vi "Lift and Clamp Test.vi"() -> ()   [LabVIEW 2014]
panel:
  in  "Clamp Direction":enum16{"Stop", "In", "Out"}(ring)
  out "Lift Encoder":T1
  in  "Lift Direction":enum16{"Stop", "Up", "Down"}(ring)
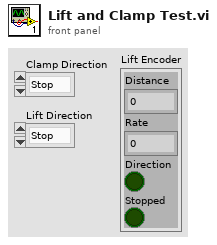
[diagram p1: front panel]
types:
  T1 = cluster{"Distance":dbl, "Rate":dbl, "Direction":bool, "Stopped":bool}
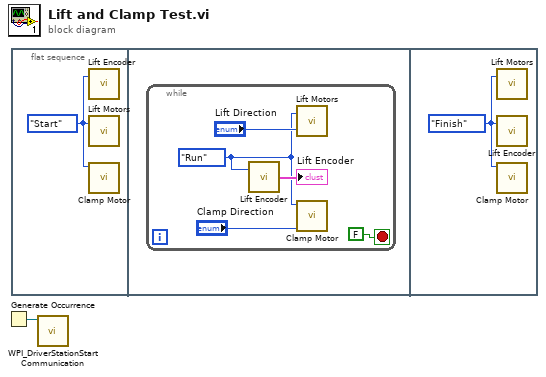
[diagram p0: block diagram]
diagram:
  n1 = Generate Occurrence() -> (w1:refnum<k4>)
  n2 = flat-sequence {
    frame #0 {
      w2 = enum8{"Start", "Run", "Finish"}."Start" ("Mode")
      n3 = call "Lift Encoder.vi"("Mode"=w2) -> ()  [unwired: 1 in, 1 out]
      n4 = call "Lift Motors.vi"("Mode"=w2) -> ()  [unwired: 2 in]
      n5 = call "Clamp Motor.vi"("Mode"=w2) -> ()  [unwired: 3 in]
    }
    frame #1 {
      n6 = while {
        stop <- FALSE stop-if-true
        w4 = enum8{"Start", "Run", "Finish"}."Run" ("Mode")
        n7 = call "Lift Encoder.vi"("Mode"=w4) -> ("Lift Encoder"=→"Lift Encoder":T1)  [unwired: 1 in]
        n8 = call "Lift Motors.vi"("Direction"="Lift Direction", "Mode"=w4) -> ()  [unwired: 1 in]
        n9 = call "Clamp Motor.vi"("Direction"="Clamp Direction", "Mode"=w4) -> ()  [unwired: 2 in]
      }
    }
    frame #2 {
      w8 = enum8{"Start", "Run", "Finish"}."Finish" ("Mode")
      n10 = call "Lift Motors.vi"("Mode"=w8) -> ()  [unwired: 2 in]
      n11 = call "Lift Encoder.vi"("Mode"=w8) -> ()  [unwired: 1 in, 1 out]
      n12 = call "Clamp Motor.vi"("Mode"=w8) -> ()  [unwired: 3 in]
    }
  }
  n13 = call <vilib>:"WPI_DriverStationStart Communication.vi"("occurrence"=w1) -> ()  [unwired: 11 in]
